vi "Convert U32 to POINT for pRes.vi"(1 "pCnt":i32=16, 2 "pRes 2":u32[](array[numeric])) -> (0 "pRes":T1[](array[typedef]))   [LabVIEW 2013, in "VRI.lvlib"]
doc: "This VI is used to convert an array of U32 to an array of POINT (pRes)."
uses:
  VRI.lvlib
  _Type Defs/Point.ctl
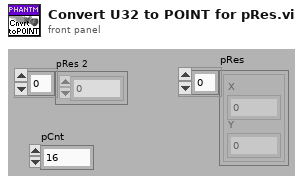
[diagram p1: front panel]
types:
  T1 = typedef "VRI.lvlib/Point.ctl" = cluster{"X":i32, "Y":i32}
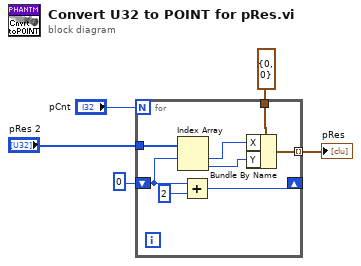
[diagram p0: block diagram]
diagram:
  n1 = for {
    N: "pCnt" -> [_]
    tunnel: "pRes 2" -> [w11]
    tunnel: T1 {"X"=0, "Y"=0} ("Point") -> [w13]
    tunnel: [w12] -> w4 mode=indexing
    shift-right: [w6] -> _
    shift-left: 0 -> [w8]
    n2 = Index Array(array=w11, index #1=w8) -> (element #1=w10:u32, element #2=w9:u32)  [unwired: 1 in]
    n3 = Add(x=w8, y=2) -> (x+y=w6:i32)
    n4 = Bundle By Name(cluster=w13, "X"=w10, "Y"=w9) -> (w12:T1)
  }
  "pRes" <- w4
